vi "S2C_PCIe7841_Proc_Close.vi"(8 "Error In":errorcluster) -> (0 "Error Out":errorcluster)   [LabVIEW 2015]
uses:
  S2C_PCIe7841_Proc_Globals.vi
  <vilib>/FPGAPlugInAG/Dynamic/niLvFpga_Close_Dynamic.vi
  <vilib>/rvi/interface/nirviCloseFPGA/nirviCloseFPGA.xnode
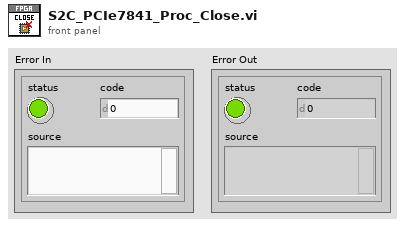
[diagram p1: front panel]
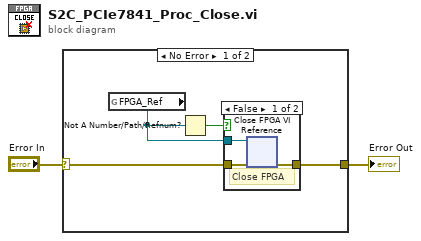
[diagram p0: block diagram]
diagram:
  n1 = case shown="No Error" "Error In" {
    selector: "Error In" -> [w6 w11]
    tunnel: [w5 w11] -> w1
    frame No Error {
      n2 = global read "S2C_PCIe7841_Proc_Globals.vi" "FPGA_Ref"() -> (w3:refnum<k20>)
      n3 = Not A Number/Path/Refnum?(number/path/refnum=w3) -> (NaN/Path/Refnum?=w4:bool)
      n4 = case shown="False" w4 {
        tunnel: w6 -> [w9 w10]
        tunnel: [w8 w10] -> w5
        tunnel: w3 -> [w7 _]
        frame False {
          # "Close FPGA"
          n5 = xnode "Close FPGA VI Reference"("FPGA VI Reference In"=w7, "error in"=w9) -> ("error out"=w8:errorcluster)
        }
        frame True {
        }
      }
    }
    frame Error {
    }
  }
  "Error Out" <- w1
